vi "Begin.vi"(8 "error in (no error)":errorcluster, 11 "Dev Elevator in":refnum<class "Dev Elevator.lvclass">) -> (0 "error out":errorcluster, 3 "Dev Elevator out":refnum<class "Dev Elevator.lvclass">)   [LabVIEW 2014, in "Dev Elevator.lvlib" / "Dev Elevator.lvclass"]
uses:
  Dev Elevator.lvclass
  Dev Elevator.lvclass/Dev Elevator.ctl
  <vilib>/Rock Robotics/WPI/Solenoid/WPI_SolenoidOpenDouble.vi
  Robot/Elevator/Elevator Class/Elevator.lvclass
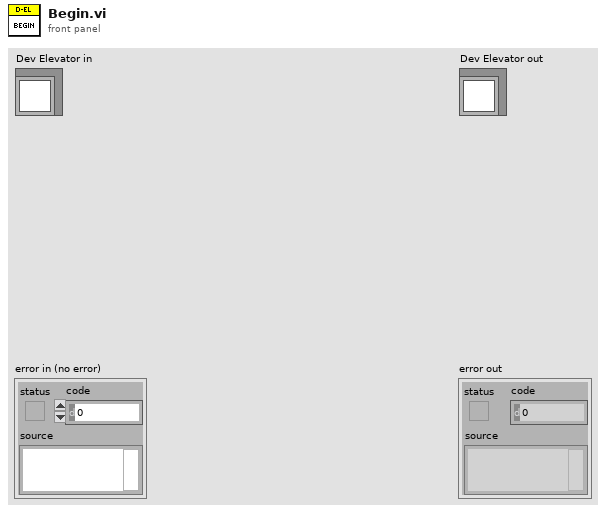
[diagram p1: front panel]
types:
  T1 = typedef "Dev Elevator.lvlib/Dev Elevator.lvclass/Dev Elevator Config.ctl" = cluster{"Brake Set Channel":T2, "Pneumatics CAN ID":u8, "Brake Release Channel":T2}
  T2 = typedef "WPI_SolenoidChannel.ctl" = enum8{"Solenoid 0", "Solenoid 1", "Solenoid 2", "Solenoid 3", "Solenoid 4", "Solenoid 5", "Solenoid 6", "Solenoid 7", "Invalid"}
  T3 = typedef "WPI_SolenoidDevRef.ctl" = cluster{"DevStatus":errorcluster, "Pneumatics Control Module":u8, "Forward Solenoid Channel":T2, "Reverse Solenoid Channel":T2}
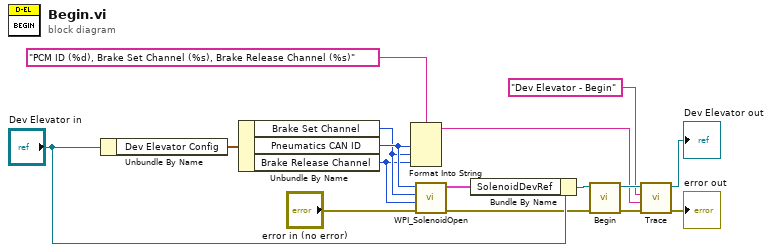
[diagram p0: block diagram]
diagram:
  n1 = Unbundle By Name("Dev Elevator in") -> ("Dev Elevator Config"=w15:T1)
  n2 = Unbundle By Name(w15) -> ("Brake Set Channel"=w2:T2, "Pneumatics CAN ID"=w3:u8, "Brake Release Channel"=w1:T2)
  n3 = Format Into String(format string="PCM ID (%d), Brake Set Channel (%s), Brake Release Channel (%s)", w3, w2, w1) -> (resulting string=w5:string)  [unwired: 2 in, 1 out]
  n4 = call-poly <vilib>:"WPI_SolenoidOpen.vi"("error in (no error)"="error in (no error)", "Reverse Solenoid Channel"=w1, "Forward Solenoid Channel"=w2, "Pneumatics Control Module (0)"=w3) -> ("error out"=w11:errorcluster, "SolenoidDevRef"=w13:T3)  [unwired: 6 in]
  n5 = Bundle By Name(cluster="Dev Elevator in", "SolenoidDevRef"=w13) -> (w14:refnum<class "Dev Elevator.lvclass">)
  n6 = call-parent "Begin.vi"("error in (no error)"=w11, "System Actor in"=w14) -> ("error out"=w8:errorcluster, "System Actor out"=w10:refnum<class "Dev Elevator.lvclass">)  [unwired: 8 in]
  n7 = call-dynamic "Trace.vi"("error in (no error)"=w8, "System Message"=w5, "System Action"="Dev Elevator - Begin", "System Actor in"=w10) -> ("error out"=→"error out":errorcluster, "System Actor out"=→"Dev Elevator out":refnum<class "Dev Elevator.lvclass">)  [unwired: 6 in]
